vi "Xbox Layout.vi"(2 "Joystick Name":string) -> (0 "Center Left":bool, 5 "Arrows":dbl, 6 "Center Right":bool, 7 "A":bool, 8 "Left Button":bool, 9 "B":bool, 10 "Right Button":bool, 11 "X":bool, 12 "L+R Throttles":dbl, 13 "Y":bool, 14 "Left Stick Y":dbl, 15 "Left Stick X":dbl, 16 "Left Stick Touch":bool, 17 "Right Stick Y":dbl, 18 "Right Stick X":dbl, 19 "Right Stick Touch":bool)   [LabVIEW 2013]
doc: "The layout of Buttons and axes from the XBOX 360 Controller"
uses:
  <vilib>/Rock Robotics/WPI/Joystick/WPI_JoystickGetSetRefNum.vi
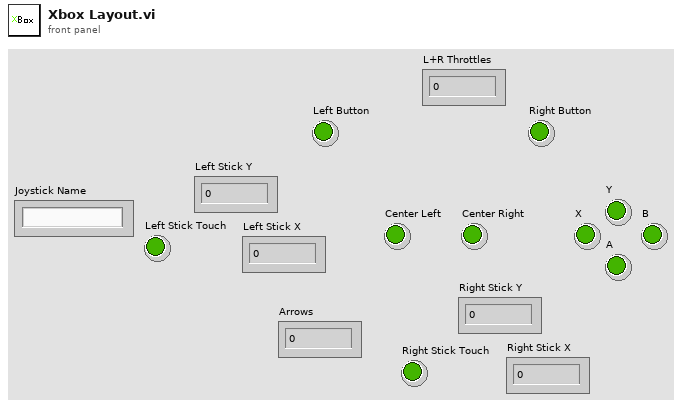
[diagram p1: front panel]
types:
  T1 = typedef "WPI_JoystickDevRef.ctl" = cluster{"Device":T2}
  T2 = typedef "WPI_JoystickDeviceEnum.ctl" = enum16{"USB 1", "USB 2", "USB 3", "USB 4", "Kinect 1", "Kinect 2"}
  T3 = typedef "WPI_JoystickButtonState.ctl" = cluster{"Button 1":bool, "Button 2":bool, "Button 3":bool, "Button 4":bool, "Button 5":bool, "Button 6":bool, "Button 7":bool, "Button 8":bool, "Button 9":bool, "Button 10":bool, "Button 11":bool, "Button 12":bool}
  T4 = cluster{"axis 1 (x)":dbl, "axis 2 (y)":dbl, "axis 3 (throttle)":dbl, "axis 4":dbl, "axis 5":dbl, "axis 6":dbl}
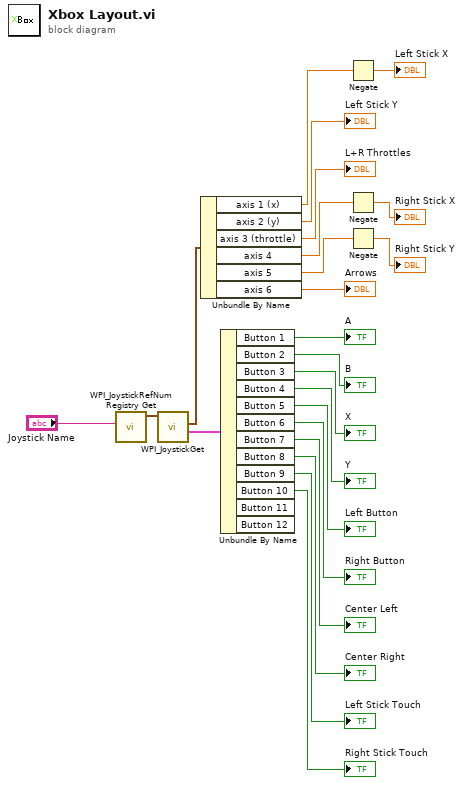
[diagram p0: block diagram]
diagram:
  n1 = call <vilib>:"WPI_JoystickRefNum Registry Get.vi"("refnum name"="Joystick Name") -> ("JoystickDevRef"=w23:T1)  [unwired: 9 in, 1 out]
  n2 = call <vilib>:"WPI_JoystickGet.vi"("JoystickDevRef"=w23) -> ("Buttons"=w21:T3, "Axes"=w20:T4)  [unwired: 4 in, 1 out]
  n3 = Unbundle By Name(w20) -> ("axis 1 (x)"=w17:dbl, "axis 2 (y)"=→"Left Stick Y":dbl, "axis 3 (throttle)"=→"L+R Throttles":dbl, "axis 4"=w16:dbl, "axis 5"=w2:dbl, "axis 6"=→"Arrows":dbl)
  n4 = Unbundle By Name(w21) -> ("Button 1"=→"A":bool, "Button 2"=→"B":bool, "Button 3"=→"X":bool, "Button 4"=→"Y":bool, "Button 5"=→"Left Button":bool, "Button 6"=→"Right Button":bool, "Button 7"=→"Center Left":bool, "Button 8"=→"Center Right":bool, "Button 9"=→"Left Stick Touch":bool, "Button 10"=→"Right Stick Touch":bool)  [unwired: 2 out]
  n5 = Negate(x=w17) -> (-x=→"Left Stick X":dbl)
  n6 = Negate(x=w16) -> (-x=→"Right Stick X":dbl)
  n7 = Negate(x=w2) -> (-x=→"Right Stick Y":dbl)
